vi "CryoCooler GUI.vi"(9 "Standalone":bool=TRUE, 10 "Init Data":variant, 11 "CryoCooler Name":string) -> ()   [LabVIEW 2021]
uses:
  typedefs/CC enum Operation Mode.ctl
  Cryo Cooler/CryoCoolerAVC/CryoCoolerAVC Command enum.ctl
  WebRelay10 Driver/CC WebRelay cluster Settings.ctl
  Subsystems/SS typedef cluster Instrument Command Queue Data.ctl
  Subsystems/SS cluster Data Queue type.ctl
  hk-channel-class/HK Item/HK Item.lvclass
  Cryo Cooler/Cryo Cooler.lvclass
  Cryo Cooler/CryoCoolerAVC/CryoCoolerAVC Command cluster.ctl
  typedefs/CC cluster Alarm Data.ctl
  CryoCooler cluster Alarm Settings.ctl
  typedefs/CC enum Status FG Action.ctl
  Cryo Cooler/CryoCoolerAVC/CryoCoolerAVC.lvclass
  C:/Development/prime/Prime-RIMAS/CryoCooler/Cryo Cooler/Cryo Cooler.lvclass
  typedefs/CC enum Subsystem Status.ctl
  Cryo Cooler/Cryo Cooler.lvclass/Cryo Cooler.ctl
  hk-channel-class/HK Item/HK Item.lvclass/HK Item.ctl
  WebRelay10 Driver/CC WebRelay enum Actions.ctl
  hk-channel-class/HK Item/HK Channel cluster Telemetry Data.ctl
  hk-channel-class/HK Item/HK Channel enum Data Type.ctl
  <vilib>/Utility/error.llb/DialogType.ctl
  Cryo Cooler/CryoCoolerAVC/CryoCoolerAVC Settings.ctl
  hk-channel-class/HK Item/Write Source.vi
  6db094d1-7fd6-4988-9962-decbce56bcaa.vi
  40afddd7-fa93-47ab-b467-3e4868690066.vi
panel:
  in  "Mode":T1
  in  "Tab Control":T2(tab)
  out "Alarm Message":string
  out "Cryo Connected":bool
  out "Alarm":bool
  in  "Status":i32[](listbox)
  out "XY Graph":T3(graph)
  out "Cryo 2":bool
  out "Cryo 1":bool
  in  "Shutdown Temp":dbl caption="Reject Temp Shutdown Temp"
  in  "Init Message":string="Connecting to Hardware..."
  in  "Reinit":bool
  out "Response":string[](array[string])
  in  "Cryo 2 Address":refnum<visa-resource-name>
  in  "Execute command":bool
  in  "Command Options":string="On"
  in  "Command":T4=1 items=["STATUS", "COOLER", "E", "ERROR", "KD", "KI", "KP", "LOGIN", "LOGOUT", "MODE", "P", "PWOUT", "SENSOR", "TC", "TEMP RJ", "TTARGET", "VERSION"]
  in  "Command 2":T4=1 items=["STATUS", "COOLER", "E", "ERROR", "KD", "KI", "KP", "LOGIN", "LOGOUT", "MODE", "P", "PWOUT", "SENSOR", "TC", "TEMP RJ", "TTARGET", "VERSION"]
  in  "Command Options 2":string="On"
  in  "Execute command 2":bool
  in  "Cryo 1 Address":refnum<visa-resource-name>
  in  "CryoCooler Type":u16(ring) items=["Simulation", "PRIME"]
  in  "Close":bool
  out "x-y":u32
  in  "Names":string[](array[string])=["USB Hub", "MACIEs", "FW Motors", "N/A", "Lesker", "ICRON Ranger", "PICO Motors", "LAN Switch", "Cryo Coolers", "HK Box"]
  in  "Refresh Button":bool
  in  "Relay Set":bool[](array[boolean]) caption="Set"
  out "Status":bool[](array[boolean])
  out "error out":errorcluster
  out "WebRelay10 Settings":T5={"Address"="", "Port"=80, "Names"=[]}
  out "Log":string
  in  "Cryo 1 Pwr":bool
  in  "Cryo 2 Pwr":bool
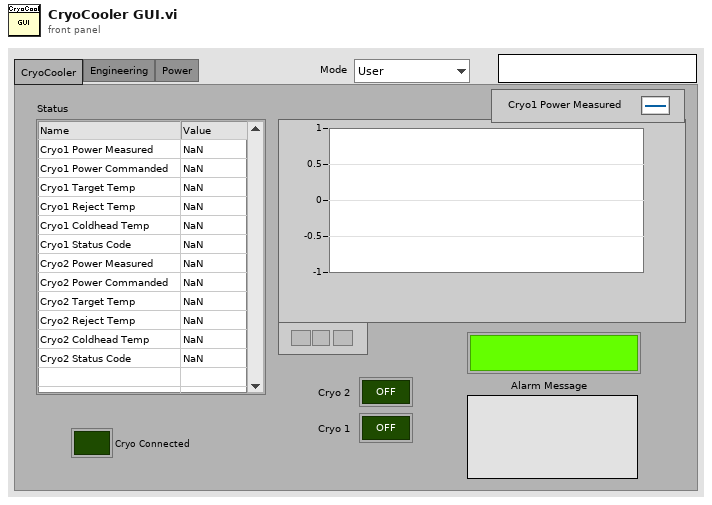
[diagram p1: front panel]
types:
  T1 = typedef "CC enum Operation Mode.ctl" = enum16{"User", "Engineering"}
  T2 = enum32{"CryoCooler", "Engineering", "Power", "Log"}
  T3 = cluster{cluster{"Time Stamp":timestamp, "Numeric":dbl}[]}[]
  T4 = typedef "CryoCoolerAVC Command enum.ctl" = u16
  T5 = typedef "CC WebRelay cluster Settings.ctl" = cluster{"Address":string, "Port":u16, "Names":string[]}
  T6 = typedef "SS typedef cluster Instrument Command Queue Data.ctl" = cluster{"Cmd":string, "Parameters":variant}
  T7 = typedef "CryoCoolerAVC Command cluster.ctl" = cluster{"Command":T4, "Options":string, "Cryo Idx":i32}
  T8 = typedef "CC cluster Alarm Data.ctl" = cluster{"Measured Value":dbl, "Alarm Low":dbl, "Alarm High":dbl, "Message":string, "Source":string}
  T9 = typedef "CryoCooler cluster Alarm Settings.ctl" = cluster{"Reject Shutdown Temp":dbl, "Reject Temp Warning":dbl, "Temperature Error Max":dbl}
  T10 = cluster{"state":refnum<user-event>, "cmd q":refnum<queue>, "Cmd":T6, "Data Q":refnum<queue>, "error":errorcluster, "next poll":timestamp, "Cryo Name":string, "poll":bool, "Channel List":refnum<class "HK Item.lvclass">[], "Focus Pos":dbl, "Cryo Cooler ref":refnum<class "Cryo Cooler.lvclass">, "Data":dbl[], "Cryo Cmd":T7, "Alarm":bool, "Alarms":T8[], "Source":string, "Cryo Alarms":T9, "Shutdown":bool}
  T11 = typedef "CC enum Status FG Action.ctl" = enum16{"Read", "Write", "Init"}
  T12 = typedef "CC enum Subsystem Status.ctl" = enum16{"Unknown", "Ready", "Error"}
  T13 = typedef "SS cluster Data Queue type.ctl" = cluster{"Source":string, "Type":string, "Data":variant}
  T14 = typedef "CC WebRelay enum Actions.ctl" = enum16{"Init", "Read Status", "Set Relay", "Close"}
  T15 = typedef "HK Item.lvclass/HK Channel enum Data Type.ctl" = enum16{"Floating Point", "Integer", "Enum", "String", "Waveform", "File"}
  T16 = typedef "HK Item.lvclass/HK Channel cluster Telemetry Data.ctl" = cluster{"Ch Names":string[], "Ch Values":dbl[], "Timestamp":timestamp, "Data Type":T15}
  T17 = typedef "CryoCoolerAVC.lvclass/CryoCoolerAVC Settings.ctl" = cluster{"CryoTek 1 Addr":refnum<visa-resource-name>, "CryoTek 2 Addr":refnum<visa-resource-name>}
  T18 = typedef "CC cluster Device Index.ctl" = cluster{"Device Type Name":string, "Curr Device Name":string, "All Instances":string[]}
  T19 = typedef "CryoCooler Default User Settings.ctl" = cluster{"Select Ch":i32[], "Default Device":string}
  T20 = typedef "HK Item.lvclass/HK Channel Units and Setup.ctl" = cluster{"Unit Type":string, "Units":string, "Configuration":string, "Digits":i32, "Data Type":T15, "Exponential?":bool, "Source":string}
  T21 = cluster{"[0]":dbl, "[1]":dbl, "[2]":dbl, "[3]":dbl, "[4]":dbl, "[5]":dbl}
  T22 = cluster{"[0]":dbl, "[1]":dbl, "[2]":dbl, "[3]":dbl, "[4]":dbl, "[5]":dbl}[]
  T23 = cluster{cluster{"Time Stamp":timestamp, "Numeric":dbl}[]}
  T24 = typedef "DialogType.ctl" = u16
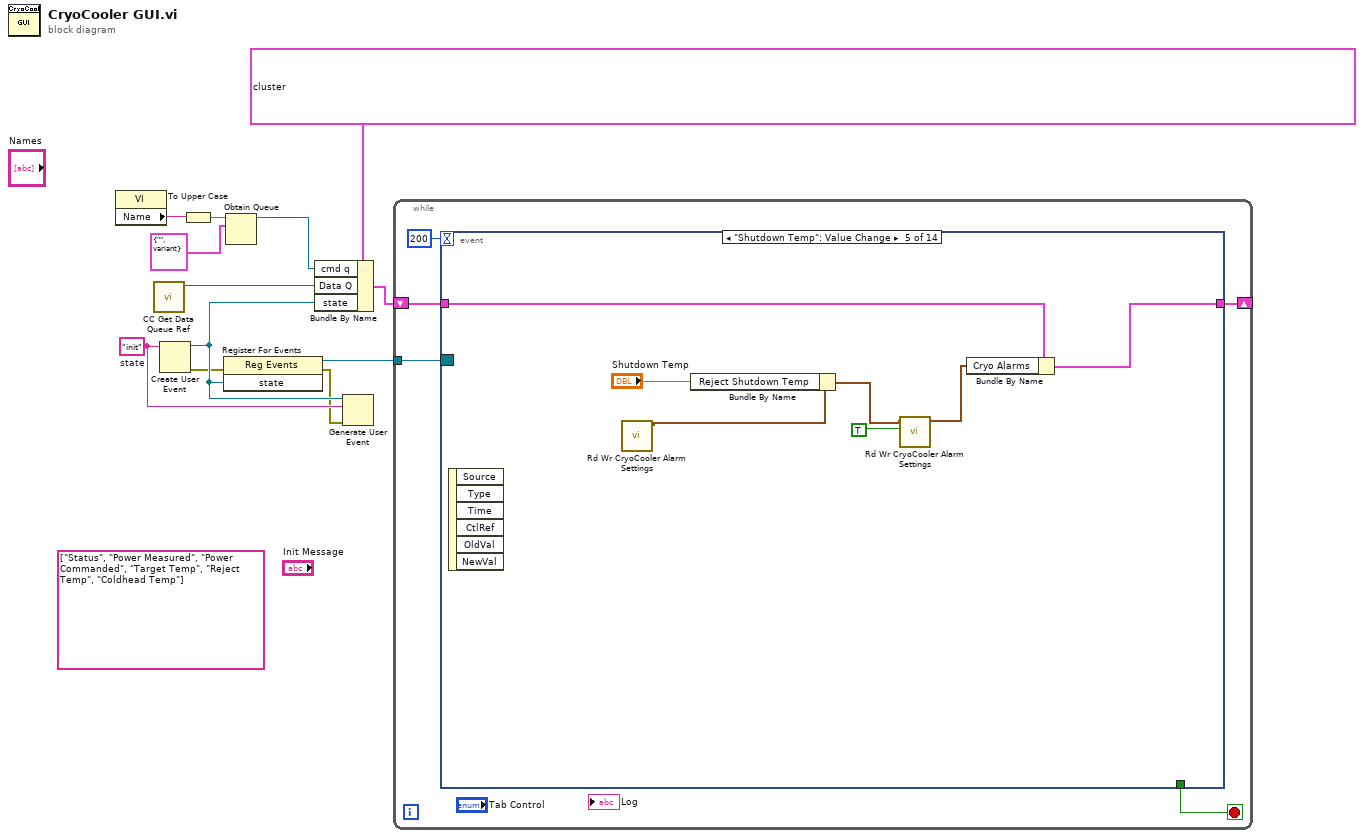
[diagram p0: block diagram]
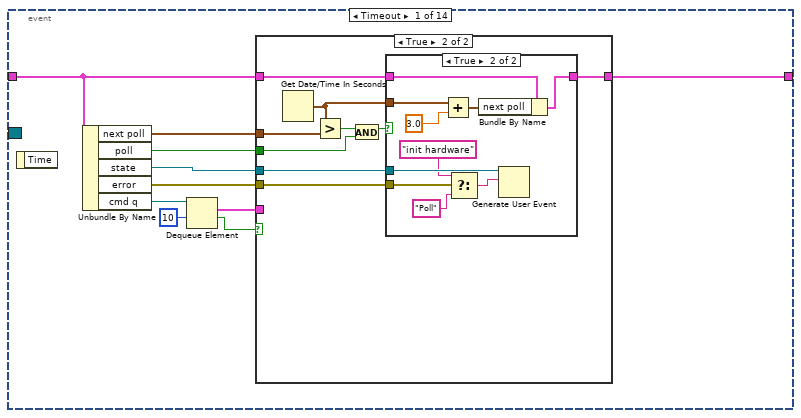
[diagram p2: hidden frame]
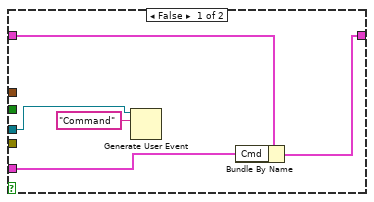
[diagram p3: hidden frame]
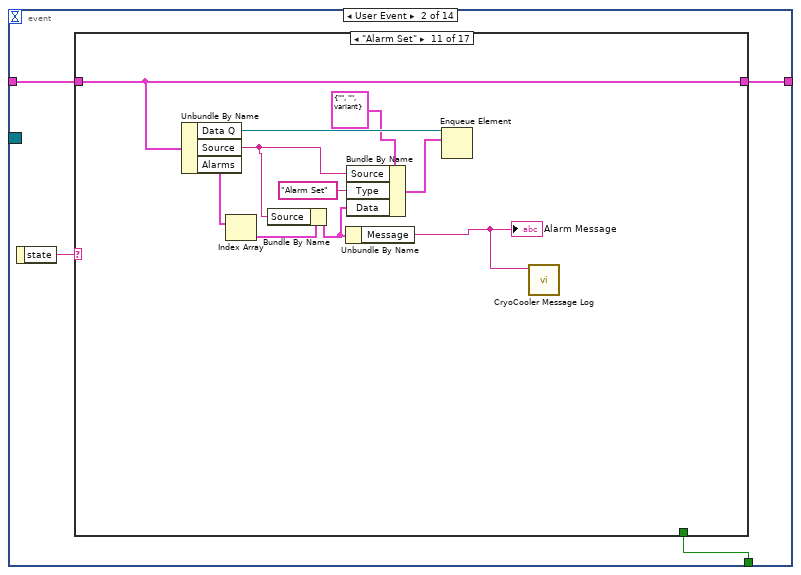
[diagram p5: hidden frame]
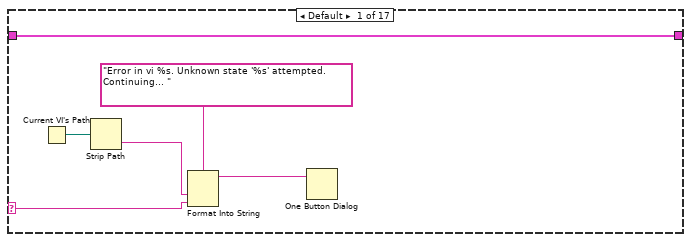
[diagram p6: hidden frame]
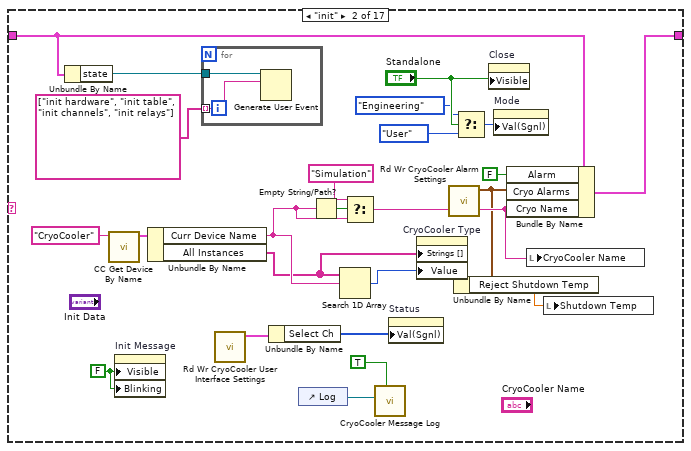
[diagram p7: hidden frame]
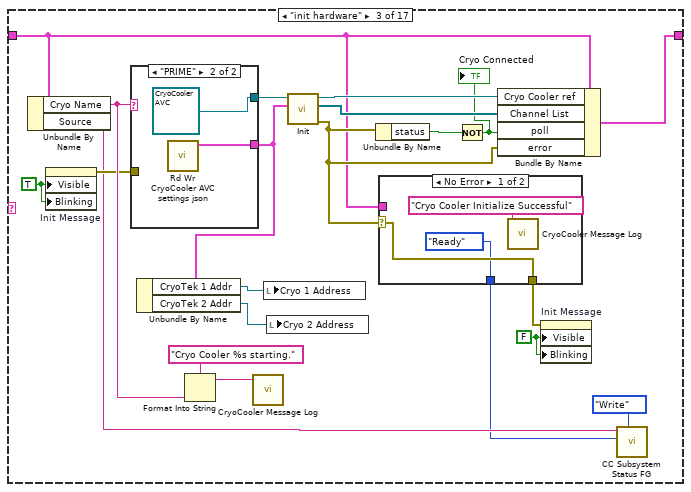
[diagram p8: hidden frame]
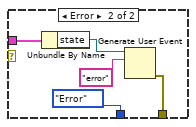
[diagram p9: hidden frame]
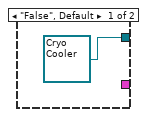
[diagram p10: hidden frame]
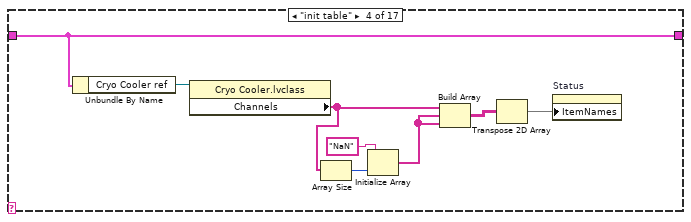
[diagram p11: hidden frame]
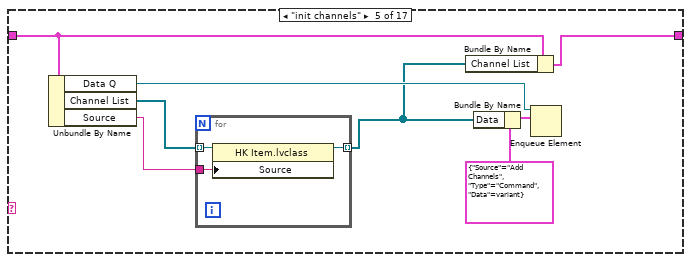
[diagram p12: hidden frame]
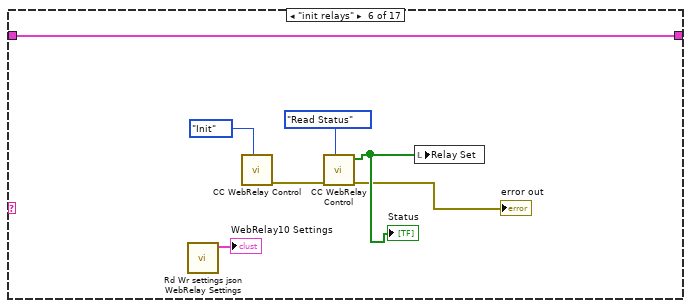
[diagram p13: hidden frame]
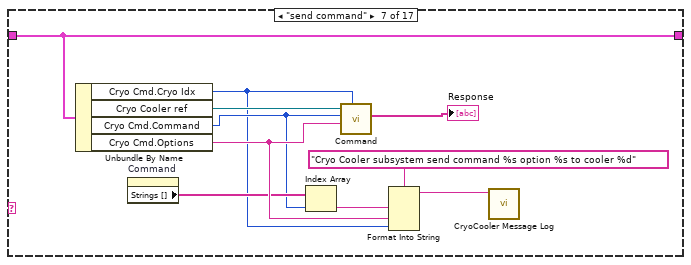
[diagram p14: hidden frame]
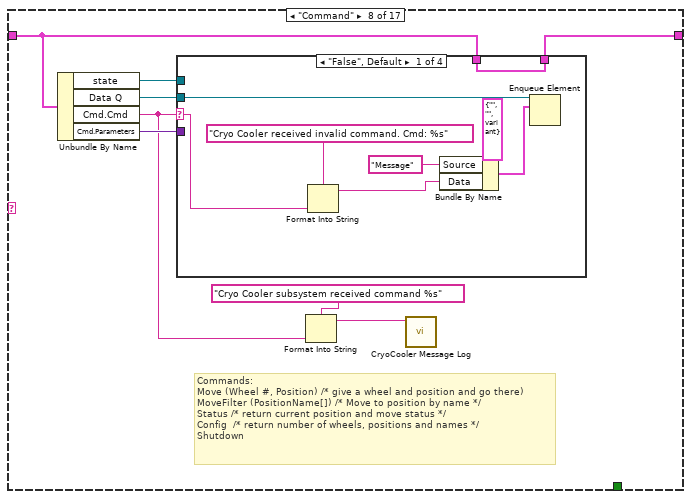
[diagram p15: hidden frame]
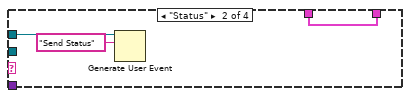
[diagram p16: hidden frame]
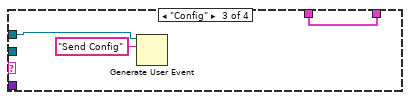
[diagram p17: hidden frame]
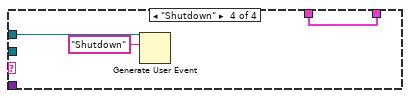
[diagram p18: hidden frame]
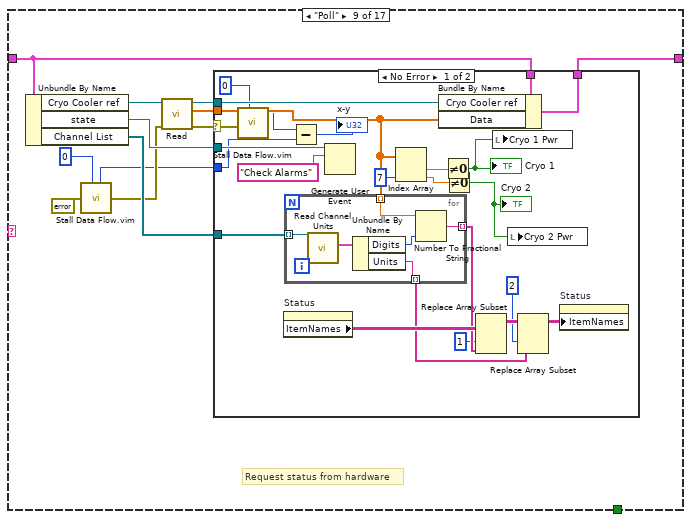
[diagram p19: hidden frame]
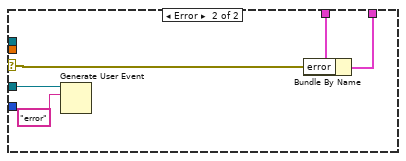
[diagram p20: hidden frame]
diagram:
  (unwired) string[] ["Status", "Power Measured", "Power Commanded", "Target Temp", "Reject Temp", "Coldhead Temp"]
  w8 = "init"  # state
  n1 = property class="VI"() -> ("Name"=w4:string)  [unwired: 2 in, 2 out]
  n2 = call "CC Get Data Queue Ref.vi"() -> ("Data Q"=w5:refnum<queue>)  [unwired: 10 in, 1 out]
  n3 = Create User Event(user event datatype=w8) -> (user event=w10:refnum<user-event>, error out=w6:errorcluster)  [unwired: 1 in]
  n4 = To Upper Case(1:w4) -> (0:w3:string)
  n5 = register-events(error in=w6, w10) -> (reference out=w9:refnum<event-registration>, error out=w7:errorcluster)  [unwired: 1 in]
  n6 = Obtain Queue(name (unnamed)=w3, element data type=T6 {"Cmd"="", "Parameters"=variant}) -> (queue out=w1:refnum<queue>)  [unwired: 3 in, 2 out]
  n7 = Bundle By Name(cluster=T10 {"state"=refnum, "cmd q"=refnum, "Cmd"={"Cmd"="", "Parameters"=variant}, "Data Q"=refnum, "error"={"status"=FALSE, "code"=0, "source"=""}, "next poll"=timestamp(0 s since 1904-01-01), "Cryo Name"="", "poll"=FALSE, "Channel List"=[], "Focus Pos"=0.0, "Cryo Cooler ref"=refnum, "Data"=[], "Cryo Cmd"={"Command"=0, "Options"="", "Cryo Idx"=0}, "Alarm"=FALSE, "Alarms"=[], "Source"="CryoCooler", "Cryo Alarms"={"Reject Shutdown Temp"=30.0, "Reject Temp Warning"=3.0, "Temperature Error Max"=60.0}, "Shutdown"=FALSE}, "cmd q"=w1, "Data Q"=w5, "state"=w10) -> (w11:T10)
  n8 = Generate User Event(user event=w10, event data cluster=w8, error in=w7) -> ()  [unwired: 1 in, 2 out]
  n9 = while {
    tunnel: w9 -> [w17]
    shift-right: [w15] -> _
    shift-left: w11 -> [w16]
    stop <- w14 stop-if-true
    n10 = event shown="[4] \"Shutdown Temp\": Value Change" {
      selector: w17 -> [_ _ _ _ _ _ _ _ _ _ _ _ _ _]
      dyn-events: _ -> [_ _ _ _ _ _ _ _ _ _ _ _ _ _]
      timeout: 200 -> [_ _ _ _ _ _ _ _ _ _ _ _ _ _]
      tunnel: w16 -> [w22 w55 w337 w346 w349 w355 w365 w377 w387 w391 w396 w417 w436 w443]
      tunnel: [w21 w54 w337 w346 w347 w355 w365 w378 w387 w391 w397 w418 w436 w443] -> w15
      tunnel: [_ w53 _ _ _ _ _ _ _ _ _ _ _ _] -> w14
      event Timeout {
        n11 = event-data() -> ()  [unwired: 1 in, 1 out]
        n12 = Unbundle By Name(w22) -> ("next poll"=w20:timestamp, "poll"=w19:bool, "state"=w23:refnum<user-event>, "error"=w18:errorcluster, "cmd q"=w27:refnum<queue>)
        n13 = Dequeue Element(queue=w27, timeout in ms (-1)=10) -> (element=w24:T6, timed out?=w25:bool)  [unwired: 1 in, 2 out]
        n14 = case shown="True" w25 {
          tunnel: w24 -> [w29 _]
          tunnel: w23 -> [w32 w38]
          tunnel: w22 -> [w30 w39]
          tunnel: [w28 w36] -> w21
          tunnel: w20 -> [_ w41]
          tunnel: w19 -> [_ w34]
          tunnel: w18 -> [_ w33]
          frame False {
            n15 = Generate User Event(user event=w32, event data cluster="Command" ("event data")) -> ()  [unwired: 2 in, 2 out]
            n16 = Bundle By Name(cluster=w30, "Cmd"=w29) -> (w28:T10)
          }
          frame True {
            n17 = Get Date/Time In Seconds() -> (seconds since 1Jan1904=w37:timestamp)
            n18 = Greater?(x=w37, y=w41) -> (0:w40:bool)
            n19 = And(x=w40, y=w34) -> (x .and. y?=w35:bool)
            n20 = case shown="True" w35 {
              tunnel: w39 -> [w42 w52]
              tunnel: w38 -> [_ w51]
              tunnel: w37 -> [_ w50]
              tunnel: [w42 w47] -> w36
              tunnel: w33 -> [_ w45]
              frame False {
              }
              frame True {
                n21 = Add(x=w50, y=3.0) -> (x+y=w48:timestamp)
                n22 = Select(t="init hardware", s=w45, f="Poll" ("event data")) -> (s? t:f=w43:string)
                n23 = Bundle By Name(cluster=w52, "next poll"=w48) -> (w47:T10)
                n24 = Generate User Event(user event=w51, event data cluster=w43) -> ()  [unwired: 2 in, 2 out]
              }
            }
          }
        }
      }
      event User Event {
        n25 = event-data() -> ("state"=w56:string)  [unwired: 1 in]
        n26 = case shown="\"Alarm Set\"" w56 {
          selector: w56 -> [w61 _ _ _ _ _ _ _ _ _ _ _ _ _ _ _ _]
          tunnel: w55 -> [w57 w84 w98 w128 w130 w146 w155 w160 w192 w240 w259 w267 w279 w297 w301 w308 w333]
          tunnel: [w57 w85 w109 w128 w131 w146 w155 w161 w193 w241 w259 w267 w279 w297 w302 w309 w333] -> w54
          tunnel: [_ _ _ _ _ _ _ _ _ _ _ _ _ _ _ _ TRUE] -> w53
          frame Default {
            n27 = Current VI's Path() -> (path=w60:path)
            n28 = Strip Path(path=w60) -> (name=w59:string)  [unwired: 1 out]
            n29 = Format Into String(format string="Error in vi %s. Unknown state '%s' attempted. Continuing... ", w59, w61) -> (resulting string=w58:string)  [unwired: 2 in, 1 out]
            n30 = One Button Dialog(message=w58) -> ()  [unwired: 1 in, 1 out]
          }
          frame "init" {
            w66 = FALSE ("Visible")
            n31 = Unbundle By Name(w84) -> ("state"=w83:refnum<user-event>)
            n32 = call "CC Get Device By Name.vi"("Device Type"="CryoCooler") -> ("Device"=w78:T18)  [unwired: 8 in, 2 out]
            n33 = property on="Init Message" class="Str"("Visible"=w66, "Blinking"=w66) -> ()  [unwired: 2 in, 2 out]
            n34 = Unbundle By Name(w78) -> ("Curr Device Name"=w77:string, "All Instances"=w76:string[])
            n35 = for {
              tunnel: w83 -> [w88]
              tunnel: string[] ["init hardware", "init table", "init channels", "init relays"] -> [w87] mode=indexing
              n36 = Generate User Event(user event=w88, event data cluster=w87) -> ()  [unwired: 2 in, 2 out]
            }
            n37 = call "Rd Wr CryoCooler User Interface Settings.vi"() -> ("Settings"=w71:T19)  [unwired: 10 in, 1 out]
            n38 = Unbundle By Name(w71) -> ("Select Ch"=w70:i32[])
            n39 = control-ref of="Log"() -> (w69:refnum<vi>)
            n40 = Empty String/Path?(string/path=w77) -> (empty?=w86:bool)
            n41 = Search 1D Array(1D array=w76, element=w77) -> (index of element=w81:i32)  [unwired: 1 in]
            n42 = Select(t="Simulation", s=w86, f=w77) -> (s? t:f=w67:string)
            n43 = call "CryoCooler Message Log.vi"("init?"=TRUE, "Log Ref"=w69) -> ()  [unwired: 8 in, 2 out]
            n44 = property on="Status" class="MCListbox (strict)"("Val(Sgnl)"=w70) -> ()  [unwired: 2 in, 2 out]
            n45 = property on="CryoCooler Type" class="Ring (strict)"("Strings []"=w76, "Value"=w81) -> ()  [unwired: 2 in, 2 out]
            n46 = call "Rd Wr CryoCooler Alarm Settings.vi"() -> ("Cryo Alarms out"=w65:T9)  [unwired: 10 in, 1 out]
            n47 = Unbundle By Name(w65) -> ("Reject Shutdown Temp"=w64:dbl)
            n48 = Select(t=CC_enum_Operation_Mode."Engineering" ("Mode"), s="Standalone", f=CC_enum_Operation_Mode."User" ("Mode")) -> (s? t:f=w72:T1)
            n49 = property on="Close" class="Bool"("Visible"="Standalone") -> ()  [unwired: 2 in, 2 out]
            n50 = property on="Mode" class="Enum (strict)"("Val(Sgnl)"=w72) -> ()  [unwired: 2 in, 2 out]
            n51 = Bundle By Name(cluster=w84, "Alarm"=FALSE, "Cryo Alarms"=w65, "Cryo Name"=w67) -> (w85:T10)
            n52 = local write "CryoCooler Name"(w67) -> ()
            n53 = local write "Shutdown Temp"(w64) -> ()
          }
          frame "init hardware" {
            w93 = FALSE ("Visible")
            w95 = TRUE ("Visible")
            n54 = Unbundle By Name(w98) -> ("Cryo Name"=w104:string, "Source"=w90:string)
            n55 = property on="Init Message" class="Str"("Visible"=w95, "Blinking"=w95) -> (error out=w94:errorcluster)  [unwired: 2 in, 1 out]
            n56 = case shown="\"PRIME\"" w104 {
              tunnel: [refnum<class "Cryo Cooler.lvclass"> refnum ("Cryo Cooler.lvclass") refnum<class "CryoCoolerAVC.lvclass"> refnum ("CryoCoolerAVC.lvclass")] -> w106
              tunnel: [_ w119] -> w103
              tunnel: w94 -> [_ _]
              frame "False", Default {
              }
              frame "PRIME" {
                n57 = call "Rd Wr CryoCooler AVC settings json.vi"() -> ("CryoCooler Settings"=w119:T17)  [unwired: 10 in, 1 out]
              }
            }
            n58 = Unbundle By Name(w103) -> ("CryoTek 1 Addr"=w102:refnum<visa-resource-name>, "CryoTek 2 Addr"=w101:refnum<visa-resource-name>)
            n59 = Format Into String(format string="Cryo Cooler %s starting.", w104) -> (resulting string=w96:string)  [unwired: 2 in, 1 out]
            n60 = call "CryoCooler Message Log.vi"("String in"=w96) -> ()  [unwired: 9 in, 2 out]
            n61 = local write "Cryo 1 Address"(w102) -> ()
            n62 = local write "Cryo 2 Address"(w101) -> ()
            n63 = call-dynamic "Init.vi"("Init Data"=w103, "Cryo Cooler in"=w106) -> ("error out"=w99:errorcluster, "Channel List"=w105:refnum<class "HK Item.lvclass">[], "Cryo Cooler out"=w107:refnum<class "Cryo Cooler.lvclass">)  [unwired: 7 in]
            n64 = Unbundle By Name(w99) -> ("status"=w108:bool)
            n65 = case shown="No Error" w99 {
              selector: w99 -> [w111 _]
              tunnel: w98 -> [_ w117]
              tunnel: [w111 w114] -> w92
              tunnel: [CC_enum_Subsystem_Status."Ready" ("Status") CC_enum_Subsystem_Status."Error" ("Status")] -> w89
              frame No Error {
                n66 = call "CryoCooler Message Log.vi"("String in"="Cryo Cooler Initialize Successful") -> ()  [unwired: 9 in, 2 out]
              }
              frame Error {
                n67 = Unbundle By Name(w117) -> ("state"=w116:refnum<user-event>)
                n68 = Generate User Event(user event=w116, event data cluster="error" ("event data")) -> (error out=w114:errorcluster)  [unwired: 2 in, 1 out]
              }
            }
            n69 = Not(x=w108) -> (.not. x?=w97:bool)
            "Cryo Connected" <- w97
            n70 = Bundle By Name(cluster=w98, "Cryo Cooler ref"=w107, "Channel List"=w105, "poll"=w97, "error"=w99) -> (w109:T10)
            n71 = property on="Init Message" class="Str"(error in=w92, "Visible"=w93, "Blinking"=w93) -> ()  [unwired: 1 in, 2 out]
            n72 = call "CC Subsystem Status FG.vi"("Action"=CC_enum_Status_FG_Action."Write", "Status"=w89, "Subsystem Name"=w90) -> ()  [unwired: 7 in, 2 out]
          }
          frame "init table" {
            n73 = Unbundle By Name(w128) -> ("Cryo Cooler ref"=w127:refnum<class "Cryo Cooler.lvclass">)
            n74 = property class="Cryo Cooler.lvclass"(reference=w127) -> ("Channels"=w125:string[])  [unwired: 1 in, 2 out]
            n75 = Array Size(array=w125) -> (size(s)=w126:i32)
            n76 = Initialize Array("NaN", w126) -> (w121:string[])
            n77 = Build Array(w125, w121, w121) -> (w123:string[][])
            n78 = Transpose 2D Array(2D array=w123) -> (transposed array=w122:string[][])
            n79 = property on="Status" class="MCListbox (strict)"("ItemNames"=w122) -> ()  [unwired: 2 in, 2 out]
          }
          frame "init channels" {
            n80 = Unbundle By Name(w130) -> ("Data Q"=w134:refnum<queue>, "Channel List"=w133:refnum<class "HK Item.lvclass">[], "Source"=w129:string)
            n81 = for {
              tunnel: w133 -> [w139] mode=indexing
              tunnel: [w138] -> w132 mode=indexing
              tunnel: w129 -> [w137]
              n82 = property class="HK Item.lvclass"(reference=w139, "Source"=w137) -> (reference out=w138:refnum<class "HK Item.lvclass">)  [unwired: 1 in, 1 out]
            }
            n83 = Bundle By Name(cluster=w130, "Channel List"=w132) -> (w131:T10)
            n84 = Bundle By Name(cluster=T13 {"Source"="Add Channels", "Type"="Command", "Data"=variant} ("element"), "Data"=w132) -> (w136:T13)
            n85 = Enqueue Element(queue=w134, element=w136) -> ()  [unwired: 2 in, 3 out]
          }
          frame "init relays" {
            n86 = call "Rd Wr settings json WebRelay Settings.vi"() -> ("WebRelay10 Settings"=→"WebRelay10 Settings":T5)  [unwired: 10 in, 1 out]
            n87 = call "CC WebRelay Control.vi"("Action"=CC_WebRelay_enum_Actions."Init") -> ("error out"=w144:errorcluster)  [unwired: 9 in, 1 out]
            n88 = call "CC WebRelay Control.vi"("Action"=CC_WebRelay_enum_Actions."Read Status", "error in (no error)"=w144) -> ("error out"=→"error out":errorcluster, "status"=w142:bool[])  [unwired: 8 in]
            "Status" <- w142
            n89 = local write "Relay Set"(w142) -> ()
          }
          frame "send command" {
            n90 = Unbundle By Name(w155) -> ("Cryo Cmd.Cryo Idx"=w147:i32, "Cryo Cooler ref"=w156:refnum<class "Cryo Cooler.lvclass">, "Cryo Cmd.Command"=w149:T4, "Cryo Cmd.Options"=w151:string)
            n91 = property on="Command" class="Ring (strict)"() -> ("Strings []"=w150:string[])  [unwired: 2 in, 2 out]
            n92 = Index Array(array=w150, index=w149) -> (element=w148:string)
            n93 = call-dynamic "Command.vi"("Cryo Idx"=w147, "Options"=w151, "Command"=w149, "Cryo Cooler in"=w156) -> ("Response"=→"Response":string[])  [unwired: 5 in, 2 out]
            n94 = Format Into String(format string="Cryo Cooler subsystem send command %s option %s to cooler %d", w148, w151, w147) -> (resulting string=w152:string)  [unwired: 2 in, 1 out]
            n95 = call "CryoCooler Message Log.vi"("String in"=w152) -> ()  [unwired: 9 in, 2 out]
          }
          frame "Command" {
            # "Commands:\nMove (Wheel #, Position) /* give a wheel and position and go there)\nMoveFilter (PositionName[]) /* Move to position by name */\nStatus /* return current position and move status */\nConfig  /* return number of wheels, positions and names */\nShutdown"
            n96 = Unbundle By Name(w160) -> ("state"=w162:refnum<user-event>, "Data Q"=w164:refnum<queue>, "Cmd.Cmd"=w158:string, "Cmd.Parameters"=w163:variant)
            n97 = case shown="\"False\", Default" w158 {
              selector: w158 -> [w166 _ _ _]
              tunnel: w164 -> [w172 _ _ _]
              tunnel: w163 -> [_ _ _ _]
              tunnel: w162 -> [_ w175 w177 w181]
              tunnel: w160 -> [w165 w173 w176 w179]
              tunnel: [w165 w173 w176 w179] -> w161
              frame "False", Default {
                n98 = Format Into String(format string="Cryo Cooler received invalid command. Cmd: %s", w166) -> (resulting string=w168:string)  [unwired: 2 in, 1 out]
                n99 = Bundle By Name(cluster=T13 {"Source"="", "Type"="", "Data"=variant} ("element"), "Source"="Message" ("Data Type"), "Data"=w168) -> (w167:T13)
                n100 = Enqueue Element(queue=w172, element=w167) -> ()  [unwired: 2 in, 3 out]
              }
              frame "Status" {
                n101 = Generate User Event(user event=w175, event data cluster="Send Status" ("event data")) -> ()  [unwired: 2 in, 2 out]
              }
              frame "Config" {
                n102 = Generate User Event(user event=w177, event data cluster="Send Config" ("event data")) -> ()  [unwired: 2 in, 2 out]
              }
              frame "Shutdown" {
                n103 = Generate User Event(user event=w181, event data cluster="Shutdown" ("event data")) -> ()  [unwired: 2 in, 2 out]
              }
            }
            n104 = Format Into String(format string="Cryo Cooler subsystem received command %s", w158) -> (resulting string=w157:string)  [unwired: 2 in, 1 out]
            n105 = call "CryoCooler Message Log.vi"("String in"=w157) -> ()  [unwired: 9 in, 2 out]
          }
          frame "Poll" {
            # "Request status from hardware"
            n106 = Unbundle By Name(w192) -> ("Cryo Cooler ref"=w190:refnum<class "Cryo Cooler.lvclass">, "state"=w191:refnum<user-event>, "Channel List"=w188:refnum<class "HK Item.lvclass">[])
            n107 = call "Stall Data Flow.vim"("value in"=errorcluster {"status"=FALSE, "code"=0, "source"=""} ("error in (no error)"), "milliseconds to wait"=u32 0) -> ("millisecond timer value"=w182:u32, "value out"=w184:errorcluster)
            n108 = call-dynamic "Read.vi"("error in (no error)"=w184, "Cryo Cooler in"=w190) -> ("error out"=w186:errorcluster, "Data"=w187:dbl[], "Cryo Cooler out"=w189:refnum<class "Cryo Cooler.lvclass">)  [unwired: 7 in]
            n109 = case shown="No Error" w186 {
              selector: w186 -> [w204 w225]
              tunnel: [w217 w224] -> w193
              tunnel: w192 -> [w216 w226]
              tunnel: w191 -> [w215 w228]
              tunnel: w189 -> [w213 _]
              tunnel: w188 -> [w212 _]
              tunnel: w187 -> [w211 _]
              tunnel: w182 -> [w201 _]
              frame No Error {
                n110 = call "Stall Data Flow.vim"("value in"=w204, "milliseconds to wait"=u32 0) -> ("millisecond timer value"=w202:u32)  [unwired: 1 out]
                n111 = property on="Status" class="MCListbox (strict)"() -> ("ItemNames"=w209:string[][])  [unwired: 2 in, 2 out]
                n112 = for {
                  tunnel: w212 -> [w223] mode=indexing
                  tunnel: w211 -> [w220] mode=indexing
                  tunnel: [w219] -> w208 mode=indexing
                  tunnel: [w218] -> w195 mode=indexing
                  n113 = call "Read Channel Units.vi"("HK Item in"=w223) -> ("Channel Setup"=w222:T20)  [unwired: 8 in, 2 out]
                  n114 = Unbundle By Name(w222) -> ("Digits"=w221:i32, "Units"=w218:string)
                  n115 = Number To Fractional String(number=w220, precision (6)=w221) -> (F-format string=w219:string)  [unwired: 2 in]
                }
                n116 = Subtract(x=w202, y=w201) -> (x-y=→"x-y":u32)
                n117 = Generate User Event(user event=w215, event data cluster="Check Alarms" ("event data")) -> ()  [unwired: 2 in, 2 out]
                n118 = Index Array(array=w211, index #2=7 ("index")) -> (element #1=w210:dbl, element #2=w205:dbl)  [unwired: 1 in]
                n119 = Bundle By Name(cluster=w216, "Cryo Cooler ref"=w213, "Data"=w211) -> (w217:T10)
                n120 = Not Equal To 0?(x=w210) -> (x != 0?=w199:bool)
                "Cryo 1" <- w199
                n121 = Not Equal To 0?(x=w205) -> (x != 0?=w198:bool)
                "Cryo 2" <- w198
                n122 = Replace Array Subset(array=w209, new element=w208, index (col)=1 ("disabled index (col)")) -> (w197:string[][])  [unwired: 1 in]
                n123 = local write "Cryo 1 Pwr"(w199) -> ()
                n124 = local write "Cryo 2 Pwr"(w198) -> ()
                n125 = Replace Array Subset(array=w197, new element=w195, index (col)=2 ("disabled index (col)")) -> (w194:string[][])  [unwired: 1 in]
                n126 = property on="Status" class="MCListbox (strict)"("ItemNames"=w194) -> ()  [unwired: 2 in, 2 out]
              }
              frame Error {
                n127 = Generate User Event(user event=w228, event data cluster="error" ("event data")) -> ()  [unwired: 2 in, 2 out]
                n128 = Bundle By Name(cluster=w226, "error"=w225) -> (w224:T10)
              }
            }
          }
          frame "Check Alarms" {
            n129 = Unbundle By Name(w240) -> ("state"=w230:refnum<user-event>, "Data"=w248:dbl[], "Alarm"=w234:bool, "Cryo Alarms"=w233:T9, "Shutdown"=w232:bool)
            n130 = Split 1D Array(array=w248, index=6) -> (first subarray=w246:dbl[], second subarray=w245:dbl[])
            n131 = Array To Cluster(array=w246) -> (cluster=w243:T21)
            n132 = Array To Cluster(array=w245) -> (cluster=w242:T21)
            n133 = Generate User Event(user event=w230, event data cluster="Send Status" ("event data")) -> ()  [unwired: 2 in, 2 out]
            n134 = Build Array(w243, w242) -> (w238:T22)
            n135 = call "CryoCooler Alarm Check.vi"("Cryo Alarms"=w233, "Array"=w238) -> ("shutdown?"=w229:bool, "Alarms"=w237:T8[], "Alarm"=w235:bool)  [unwired: 6 in, 1 out]
            "Alarm" <- w235
            n136 = Compound Arithmetic op=AND(w235, invert w234) -> (w239:bool)
            n137 = Compound Arithmetic op=AND(w234, invert w235) -> (w236:bool)
            n138 = Compound Arithmetic op=AND(w229, invert w232) -> (w231:bool)
            n139 = case shown="True" w239 {
              tunnel: w230 -> [_ w254]
              frame False {
              }
              frame True {
                n140 = Generate User Event(user event=w254, event data cluster="Alarm Set" ("event data")) -> ()  [unwired: 2 in, 2 out]
              }
            }
            n141 = case shown="True" w236 {
              tunnel: w230 -> [_ w252]
              frame False {
              }
              frame True {
                n142 = Generate User Event(user event=w252, event data cluster="Alarm Clear" ("event data")) -> ()  [unwired: 2 in, 2 out]
              }
            }
            n143 = case shown="True" w231 {
              tunnel: w230 -> [_ w250]
              frame False {
              }
              frame True {
                n144 = Generate User Event(user event=w250, event data cluster="Alarm Shutdown" ("event data")) -> ()  [unwired: 2 in, 2 out]
              }
            }
            n145 = Bundle By Name(cluster=w240, "Shutdown"=w229, "Alarm"=w235, "Alarms"=w237) -> (w241:T10)
          }
          frame "Alarm Set" {
            n146 = Unbundle By Name(w259) -> ("Data Q"=w264:refnum<queue>, "Source"=w256:string, "Alarms"=w261:T8[])
            n147 = Index Array(array=w261) -> (element=w260:T8)  [unwired: 1 in]
            n148 = Bundle By Name(cluster=w260, "Source"=w256) -> (w257:T8)
            n149 = Unbundle By Name(w257) -> ("Message"=w258:string)
            "Alarm Message" <- w258
            n150 = Bundle By Name(cluster=T13 {"Source"="", "Type"="", "Data"=variant} ("element"), "Source"=w256, "Type"="Alarm Set", "Data"=w257) -> (w255:T13)
            n151 = Enqueue Element(queue=w264, element=w255) -> ()  [unwired: 2 in, 3 out]
            n152 = call "CryoCooler Message Log.vi"("String in"=w258) -> ()  [unwired: 9 in, 2 out]
          }
          frame "Alarm Clear" {
            n153 = Unbundle By Name(w267) -> ("Data Q"=w271:refnum<queue>, "Source"=w268:string)
            n154 = Bundle By Name(cluster=T13 {"Source"="", "Type"="", "Data"=variant} ("element"), "Source"=w268, "Type"="Alarm Clear") -> (w265:T13)
            n155 = call "CryoCooler Message Log.vi"("String in"="Alarm condition cleared.") -> ()  [unwired: 9 in, 2 out]
            n156 = Enqueue Element(queue=w271, element=w265) -> ()  [unwired: 2 in, 3 out]
          }
          frame "Alarm Shutdown" {
            w274 = "Off"
            w273 = T4 1 items=["STATUS", "COOLER", "E", "ERROR", "KD", "KI", "KP", "LOGIN", "LOGOUT", "MODE", "P", "PWOUT", "SENSOR", "TC", "TEMP RJ", "TTARGET", "VERSION"] ("Cryo Cmd.Command")
            n157 = Unbundle By Name(w279) -> ("Cryo Cooler ref"=w280:refnum<class "Cryo Cooler.lvclass">)
            n158 = call-dynamic "Command.vi"("Cryo Idx"=0, "Options"=w274, "Command"=w273, "Cryo Cooler in"=w280) -> ("error out"=w272:errorcluster, "Cryo Cooler out"=w277:refnum<class "Cryo Cooler.lvclass">)  [unwired: 5 in, 1 out]
            n159 = call-dynamic "Command.vi"("Cryo Idx"=1, "error in (no error)"=w272, "Options"=w274, "Command"=w273, "Cryo Cooler in"=w277) -> ()  [unwired: 4 in, 3 out]
            n160 = call "CryoCooler Message Log.vi"("String in"="Cryo Cooler reject temperature too high. Turning off Cryo Coolers.") -> ()  [unwired: 9 in, 2 out]
          }
          frame "Send Status" {
            n161 = Unbundle By Name(w297) -> ("Data Q"=w296:refnum<queue>, "Source"=w281:string, "Cryo Cooler ref"=w289:refnum<class "Cryo Cooler.lvclass">, "Data"=w286:dbl[])
            n162 = Get Date/Time In Seconds() -> (seconds since 1Jan1904=w287:timestamp)
            n163 = call "Read Channels.vi"("Cryo Cooler in"=w289) -> ("Channels"=w288:string[])  [unwired: 8 in, 2 out]
            n164 = Bundle(cluster=T16 {"Ch Names"=[], "Ch Values"=[], "Timestamp"=timestamp(0 s since 1904-01-01), "Data Type"=enum."Floating Point"}, "Ch Names"=w288, "Ch Values"=w286, "Timestamp"=w287, "Data Type"=HK_Channel_enum_Data_Type."Floating Point") -> (w291:T16)
            n165 = call "CC CryoCooler Data buffer.vi"("Write?"=TRUE, "Data"=w286, "Time Stamp"=w287) -> ("XY Graph"=w283:T3)  [unwired: 7 in, 1 out]
            n166 = for {
              tunnel: "Status" -> [w299] mode=indexing
              tunnel: w283 -> [w300]
              tunnel: [w298] -> w282 mode=indexing
              n167 = Index Array(array=w300, index=w299) -> (element=w298:T23)
            }
            "XY Graph" <- w282
            n168 = Bundle By Name(cluster=T13 {"Source"="", "Type"="", "Data"=variant} ("element"), "Source"=w281, "Type"="Floating Point" ("Data Type"), "Data"=w291) -> (w293:T13)
            n169 = Enqueue Element(queue=w296, element=w293) -> ()  [unwired: 2 in, 3 out]
          }
          frame "Reinit" {
            n170 = Unbundle By Name(w301) -> ("Cryo Cooler ref"=w305:refnum<class "Cryo Cooler.lvclass">, "state"=w307:refnum<user-event>)
            n171 = call-dynamic "Close.vi"("Cryo Cooler in"=w305) -> ("error out"=w304:errorcluster, "Cryo Cooler out"=w303:refnum<class "Cryo Cooler.lvclass">)  [unwired: 9 in]
            n172 = Generate User Event(user event=w307, event data cluster="init hardware" ("event data")) -> ()  [unwired: 2 in, 2 out]
            n173 = call <vilib>:"Clear Errors.vi"("error in (no error)"=w304) -> ()  [unwired: 5 in, 2 out]
            n174 = Bundle By Name(cluster=w301, "Cryo Cooler ref"=w303) -> (w302:T10)
          }
          frame "error" {
            w321 = T24 0 items=["no dialog", "OK message", "continue or stop message", "OK message + warnings", "continue/stop + warnings"] ("type of dialog (OK msg:1)")
            n175 = Unbundle By Name(w308) -> ("Cryo Name"=w313:string, "error"=w324:errorcluster, "error.code"=w327:i32, "error.source"=w325:string, "Data Q"=w315:refnum<queue>)
            n176 = call <vilib>:"Simple Error Handler.vi"("type of dialog (OK msg:1)"=w321, "error in (no error)"=w324) -> ("message"=w323:string)  [unwired: 3 in, 4 out]
            n177 = Bundle By Name(cluster=T8 {"Measured Value"=0.0, "Alarm Low"=0.0, "Alarm High"=0.0, "Message"="", "Source"=""} ("element"), "Source"=w313, "Message"="CryoCooler Initialization Error. Check Communications port.") -> (w317:T8)
            n178 = Format Into String(format string="Error from Cryo Cooler \"%s\". Error # %d, Error Source: %s, Error message \"%s\"", w313, w327, w325, w323) -> (resulting string=w322:string)  [unwired: 2 in, 1 out]
            n179 = Bundle By Name(cluster=T13 {"Source"="", "Type"="", "Data"=variant} ("element"), "Source"=w313, "Type"="Alarm Set", "Data"=w317) -> (w314:T13)
            n180 = call "CryoCooler Message Log.vi"("String in"=w322) -> ()  [unwired: 9 in, 2 out]
            n181 = Get Date/Time In Seconds() -> (seconds since 1Jan1904=w312:timestamp)
            n182 = Add(x=w312, y=120.0) -> (x+y=w310:timestamp)
            n183 = Enqueue Element(queue=w315, element=w314) -> ()  [unwired: 2 in, 3 out]
            n184 = Bundle By Name(cluster=w308, "next poll"=w310) -> (w309:T10)
          }
          frame "Shutdown" {
            n185 = Unbundle By Name(w333) -> ("Data Q"=w332:refnum<queue>, "Cryo Cooler ref"=w331:refnum<class "Cryo Cooler.lvclass">)
            n186 = call-dynamic "Close.vi"("Cryo Cooler in"=w331) -> ("error out"=w330:errorcluster)  [unwired: 9 in, 1 out]
            n187 = Release Queue(queue=w332) -> ()  [unwired: 2 in, 3 out]
            n188 = call <vilib>:"Clear Errors.vi"("error in (no error)"=w330) -> ()  [unwired: 5 in, 2 out]
            n189 = call "CC WebRelay Control.vi"("Action"=CC_WebRelay_enum_Actions."Close") -> ()  [unwired: 9 in, 2 out]
            n190 = call "CryoCooler Message Log.vi"("String in"="CryoCooler shutting down.") -> ()  [unwired: 9 in, 2 out]
          }
        }
      }
      event "Refresh Button": Value Change {
        n191 = event-data() -> ()  [unwired: 1 in, 6 out]
        n192 = call "CC WebRelay Control.vi"("Action"=CC_WebRelay_enum_Actions."Read Status") -> ("status"=w335:bool[])  [unwired: 9 in, 1 out]
        n193 = local write "Relay Set"(w335) -> ()
      }
      event "Relay Set": Value Change {
        n194 = event-data() -> ("OldVal"=w344:bool[], "NewVal"=w340:bool[])  [unwired: 1 in]
        n195 = Not Equal?(x=w344, y=w340) -> (x != y?=w343:bool[])
        n196 = Search 1D Array(1D array=w343, element=TRUE) -> (index of element=w339:i32)  [unwired: 1 in]
        n197 = Increment(x=w339) -> (x+1=w341:i32)
        n198 = Index Array(array=w340, index=w339) -> (element=w338:bool)
        n199 = call "CC WebRelay Control.vi"("Action"=CC_WebRelay_enum_Actions."Set Relay", "state"=w338, "Relay (1 to 10)"=w341) -> ()  [unwired: 7 in, 2 out]
      }
      event "Shutdown Temp": Value Change {
        n200 = event-data() -> ()  [unwired: 1 in, 6 out]
        n201 = call "Rd Wr CryoCooler Alarm Settings.vi"() -> ("Cryo Alarms out"=w352:T9)  [unwired: 10 in, 1 out]
        n202 = Bundle By Name(cluster=w352, "Reject Shutdown Temp"="Shutdown Temp") -> (w351:T9)
        n203 = call "Rd Wr CryoCooler Alarm Settings.vi"("Write? (F:Read)"=TRUE, "Cryo Alarms"=w351) -> ("Cryo Alarms out"=w348:T9)  [unwired: 8 in, 1 out]
        n204 = Bundle By Name(cluster=w349, "Cryo Alarms"=w348) -> (w347:T10)
      }
      event "Standalone": Value Change {
        n205 = event-data() -> ("NewVal"=w354:bool)  [unwired: 1 in, 5 out]
        n206 = property on="Close" class="Bool"("Visible"=w354) -> ()  [unwired: 2 in, 2 out]
      }
      event "Status": Value Change {
        n207 = event-data() -> ("NewVal"=w358:i32[])  [unwired: 1 in]
        n208 = call "CC CryoCooler Data buffer.vi"() -> ("XY Graph"=w362:T3)  [unwired: 10 in, 1 out]
        n209 = call "Rd Wr CryoCooler User Interface Settings.vi"() -> ("Settings"=w359:T19)  [unwired: 10 in, 1 out]
        n210 = for {
          tunnel: w358 -> [w367] mode=indexing
          tunnel: w362 -> [w368]
          tunnel: [w366] -> w361 mode=indexing
          n211 = Index Array(array=w368, index=w367) -> (element=w366:T23)
        }
        n212 = Bundle By Name(cluster=w359, "Select Ch"=w358) -> (w357:T19)
        n213 = Unbundle By Name(w365) -> ("Cryo Cooler ref"=w364:refnum<class "Cryo Cooler.lvclass">)
        n214 = property class="Cryo Cooler.lvclass"(reference=w364) -> ("Channels"=w363:string[])  [unwired: 1 in, 2 out]
        n215 = call "Rd Wr CryoCooler User Interface Settings.vi"("Write? (F:Read)"=TRUE, "Settings"=w357) -> ()  [unwired: 8 in, 2 out]
        n216 = property on="XY Graph" class="XYGraph (strict)"("Value"=w361) -> (error out=w360:errorcluster)  [unwired: 2 in, 1 out]
        n217 = for {
          N -> [w370]
          tunnel: w358 -> [w373] mode=indexing
          tunnel: w363 -> [w374]
          tunnel: w360 -> [w369]
          i -> [w372]
          n218 = Index Array(array=w374, index=w373) -> (element=w371:string)
          n219 = property on="XY Graph" class="XYGraph (strict)"(error in=w369, "Active Plot"=w372, "Plot.Plot Name"=w371, "LegNumRows"=w370) -> ()  [unwired: 1 in, 2 out]
        }
      }
      event "CryoCooler Type": Value Change {
        n220 = event-data() -> ("CtlRef"=w382:refnum<vi>)  [unwired: 1 in, 5 out]
        n221 = property class="Ring (strict)"(reference=w382) -> ("Strings []"=w381:string[])  [unwired: 1 in, 2 out]
        n222 = Unbundle By Name(w377) -> ("state"=w376:refnum<user-event>)
        n223 = Generate User Event(user event=w376, event data cluster="Reinit" ("event data")) -> ()  [unwired: 2 in, 2 out]
        n224 = Index Array(array=w381, index="CryoCooler Type") -> (element=w379:string)
        n225 = Bundle By Name(cluster=w377, "Cryo Name"=w379) -> (w378:T10)
      }
      event "Cryo 1 Address", "Cryo 2 Address": Value Change {
        n226 = event-data() -> ()  [unwired: 1 in, 6 out]
        n227 = Unbundle By Name(w387) -> ("state"=w386:refnum<user-event>)
        n228 = Bundle By Name(cluster=T17 {"CryoTek 1 Addr"="", "CryoTek 2 Addr"=""} ("CryoCooler Settings"), "CryoTek 1 Addr"="Cryo 1 Address", "CryoTek 2 Addr"="Cryo 2 Address") -> (w383:T17)
        n229 = Generate User Event(user event=w386, event data cluster="Reinit" ("event data")) -> ()  [unwired: 2 in, 2 out]
        n230 = call "Rd Wr CryoCooler AVC settings json.vi"("Write? (F:Read)"=TRUE, "CryoCooler Settings"=w383) -> ()  [unwired: 8 in, 2 out]
      }
      event "Reinit": Value Change {
        n231 = event-data() -> ()  [unwired: 1 in, 6 out]
        n232 = Unbundle By Name(w391) -> ("state"=w393:refnum<user-event>)
        n233 = Generate User Event(user event=w393, event data cluster="Reinit" ("event data")) -> ()  [unwired: 2 in, 2 out]
      }
      event "Execute command", "Execute command 2": Value Change {
        n234 = event-data() -> ("CtlRef"=w405:refnum<vi>)  [unwired: 1 in]
        n235 = property class="Bool"(reference=w405) -> ("Label.Text"=w404:string)  [unwired: 1 in, 2 out]
        n236 = Unbundle By Name(w396) -> ("state"=w395:refnum<user-event>)
        n237 = Match Pattern(string=w404, regular expression=".*2") -> (offset past match=w402:i32)  [unwired: 1 in, 3 out]
        n238 = Generate User Event(user event=w395, event data cluster="send command" ("event data")) -> ()  [unwired: 2 in, 2 out]
        n239 = Less Than 0?(x=w402) -> (x < 0?=w401:bool)
        n240 = case shown="False" w401 {
          tunnel: ["Command 2" "Command"] -> w399
          tunnel: ["Command Options 2" "Command Options"] -> w398
          tunnel: [1 0] -> w400
          frame False {
          }
          frame True {
          }
        }
        n241 = Bundle By Name(cluster=w396, "Cryo Cmd.Cryo Idx"=w400, "Cryo Cmd.Command"=w399, "Cryo Cmd.Options"=w398) -> (w397:T10)
      }
      event "Cryo 1 Pwr", "Cryo 2 Pwr": Value Change {
        w426 = T4 1 items=["STATUS", "COOLER", "E", "ERROR", "KD", "KI", "KP", "LOGIN", "LOGOUT", "MODE", "P", "PWOUT", "SENSOR", "TC", "TEMP RJ", "TTARGET", "VERSION"] ("Cryo Cmd.Command")
        n242 = event-data() -> ("CtlRef"=w419:refnum<vi>)  [unwired: 1 in]
        n243 = property class="Bool (strict)"(reference=w419) -> ("Label.Text"=w422:string)  [unwired: 1 in, 2 out]
        n244 = Unbundle By Name(w417) -> ("state"=w428:refnum<user-event>)
        n245 = Match Pattern(string=w422, regular expression=".*2") -> (offset past match=w420:i32)  [unwired: 1 in, 3 out]
        n246 = Less Than 0?(x=w420) -> (x < 0?=w416:bool)
        n247 = Generate User Event(user event=w428, event data cluster="send command" ("event data")) -> ()  [unwired: 2 in, 2 out]
        n248 = case shown="False" w416 {
          tunnel: "Cryo 1 Pwr" -> [_ w432]
          tunnel: [w430 w432] -> w414
          tunnel: [1 0] -> w413
          tunnel: "Cryo 2 Pwr" -> [w430 _]
          frame False {
          }
          frame True {
          }
        }
        n249 = Select(t="On", s=w414, f="Off") -> (s? t:f=w423:string)
        n250 = Bundle By Name(cluster=w417, "Cryo Cmd.Command"=w426, "Cryo Cmd.Options"=w423, "Cryo Cmd.Cryo Idx"=w413) -> (w418:T10)
      }
      event Value Change {
        n251 = event-data() -> ()  [unwired: 1 in, 6 out]
        n252 = case shown="\"User\", Default" "Mode" {
          tunnel: [bool[] [TRUE, FALSE, FALSE] bool[] [TRUE, TRUE, TRUE]] -> w433
          frame "User", Default {
          }
          frame "Engineering" {
          }
        }
        n253 = property on="Tab Control" class="TabCtl (strict)"() -> ("Pages"=w434:refnum<vi>[])  [unwired: 2 in, 2 out]
        n254 = for {
          tunnel: w434 -> [w438] mode=indexing
          tunnel: w433 -> [w437] mode=indexing
          n255 = property class="Page"(reference=w438, "PageVis"=w437) -> ()  [unwired: 1 in, 2 out]
        }
      }
      event "Close": Value Change {
        n256 = event-data() -> ()  [unwired: 1 in, 2 out]
        n257 = Unbundle By Name(w443) -> ("state"=w442:refnum<user-event>)
        n258 = Generate User Event(user event=w442, event data cluster="Shutdown" ("event data")) -> ()  [unwired: 2 in, 2 out]
      }
    }
  }
